vi "Set Item by key.vi"(8 "error in (no error)":errorcluster caption="错误输入（无错误）", 9 "Value":variant, 10 "Key":variant, 11 "HashTable 输入":refnum<class "HashTable.lvclass"> caption="DNL_LabVIEW Object in") -> (0 "error out":errorcluster caption="错误输出", 3 "HashTable 输出":refnum<class "HashTable.lvclass"> caption="DNL_LabVIEW Object out")   [LabVIEW 2012, in "HashTable.lvclass"]
uses:
  HashTable.lvclass
  HashTable.lvclass/HashTable.ctl
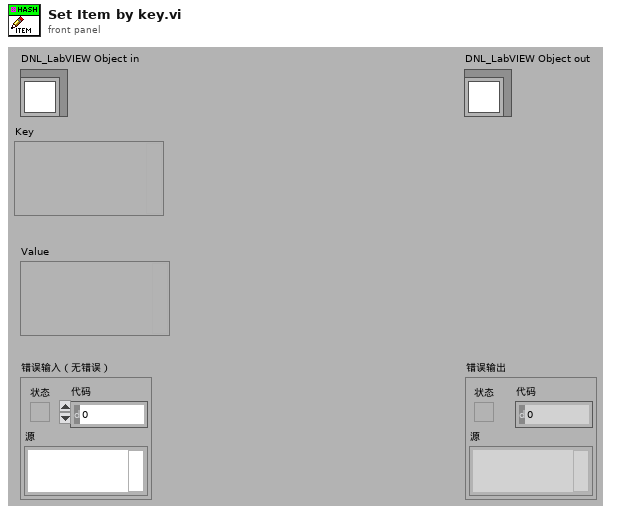
[diagram p1: front panel]
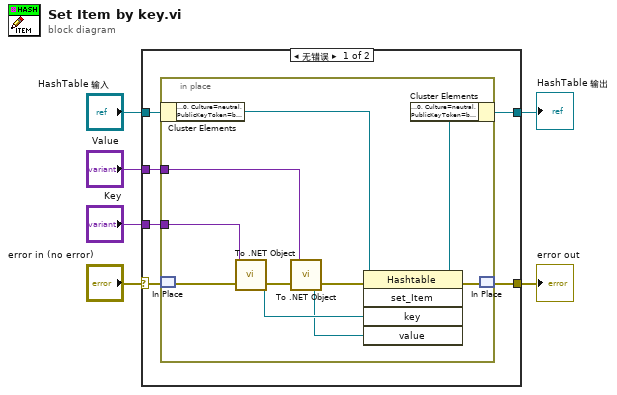
[diagram p0: block diagram]
diagram:
  n1 = case shown="无错误" "error in (no error)" {
    selector: "error in (no error)" -> [w10 w24]
    tunnel: [w9 w24] -> w5
    tunnel: [w11 w23] -> w3
    tunnel: "HashTable 输入" -> [w12 w23]
    tunnel: "Value" -> [w8 _]
    tunnel: "Key" -> [w7 _]
    frame No Error {
      n2 = in-place {
        in-place-border: w8 -> [w14]
        in-place-border: w7 -> [w13]
        n3 = in-place-cluster #1(w12) -> ("HashTable"=w22:refnum<k24>)
        n4 = in-place-match #2(w10) -> (w20:errorcluster)
        n5 = call <vilib>:"To .NET Object.vi"("error in (no error)"=w20, "anything"=w13) -> ("error out"=w18:errorcluster, ".NET object"=w19:refnum<k24>)
        n6 = call <vilib>:"To .NET Object.vi"("error in (no error)"=w18, "anything"=w14) -> ("error out"=w17:errorcluster, ".NET object"=w16:refnum<k24>)
        n7 = invoke class="Hashtable" method="set_Item"(reference=w22, error in=w17, "key"=w19, "value"=w16) -> (reference out=w21:refnum<k24>, error out=w15:errorcluster)  [unwired: 1 in, 3 out]
        n8 = in-place-cluster #1("HashTable"=w21) -> (w11:refnum<class "HashTable.lvclass">)
        n9 = in-place-match #2(w15) -> (w9:errorcluster)
      }
    }
    frame Error {
    }
  }
  "error out" <- w5
  "HashTable 输出" <- w3
